vi "draw1.vi"(0 "new position":cluster{"x":i16, "y":i16}, 1 "L 1":dbl(slide)=80.0 scale=0.0..200.0, 2 "L 2":dbl(slide)=80.0 scale=0.0..200.0, 3 "Angle1":dbl(knob)=-45.83837436417874 scale=-90.0..90.0, 4 "Angle 2":dbl(knob)=-72.06882847083946 scale=-90.0..90.0, 5 "input pic in loop":picture, 7 "bias":dbl) -> (14 "end effector":cluster{dbl, dbl}={159.01647214211073, 1.9100783062530127} {"?" format="%.1f"; "?" format="%#.1f"}, 15 "mag":dbl, 16 "angle":dbl, 17 "2D Picture":picture, 18 "shift pic":picture)   [LabVIEW 2024]
panel:
  # "A 2"
  # "L1"
  # "L2"
  # "A 1"
  # "mm"
  # "mm"
  # "mm"
  # "mm"
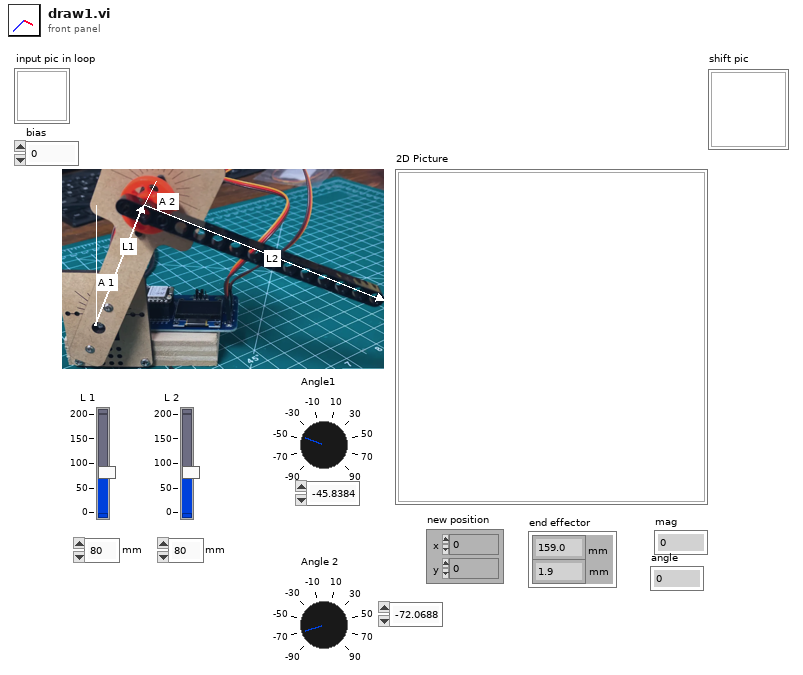
[diagram p1: front panel]
types:
  T1 = cluster{"Width":u16, "Style":enum32{"Solid", "Dash", "Dot", "DashDot", "DashDotDot"}}
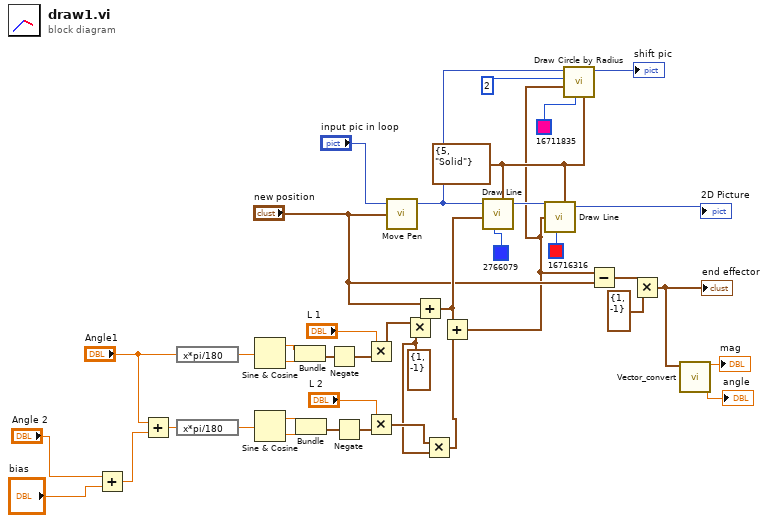
[diagram p0: block diagram]
diagram:
  w1 = cluster{"x":i16, "y":i16} {"x"=1, "y"=-1} ("new position")
  w15 = T1 {"Width"=5, "Style"=enum."Solid"} ("pen")
  n1 = Add(x="Angle 2", y="bias") -> (x+y=w8:dbl)
  n2 = Add(x="Angle1", y=w8) -> (x+y=w32:dbl)
  n3 = expression code="x*pi/180"("Angle1") -> (w40:dbl)
  n4 = expression code="x*pi/180"(w32) -> (w37:dbl)
  n5 = Sine & Cosine(0:w40) -> (1:w25:dbl, 2:w24:dbl)
  n6 = Sine & Cosine(0:w37) -> (1:w22:dbl, 2:w21:dbl)
  n7 = Bundle(w25, w24) -> (w39:cluster{dbl, dbl})  [unwired: 1 in]
  n8 = Bundle(w22, w21) -> (w38:cluster{dbl, dbl})  [unwired: 1 in]
  n9 = Negate(x=w39) -> (-x=w23:cluster{dbl, dbl})
  n10 = Negate(x=w38) -> (-x=w20:cluster{dbl, dbl})
  n11 = Multiply(x="L 1", y=w23) -> (x*y=w5:cluster{dbl, dbl})
  n12 = Multiply(x="L 2", y=w20) -> (x*y=w2:cluster{dbl, dbl})
  n13 = call <vilib>:"Move Pen.vi"("new position"="new position", "picture"="input pic in loop") -> ("new picture"=w13:picture)  [unwired: 3 in]
  n14 = Multiply(x=w5, y=w1) -> (x*y=w4:cluster{dbl, dbl})
  n15 = Add(x="new position", y=w4) -> (x+y=w35:cluster{dbl, dbl})
  n16 = Multiply(x=w2, y=w1) -> (x*y=w3:cluster{dbl, dbl})
  n17 = Add(x=w3, y=w35) -> (x+y=w14:cluster{dbl, dbl})
  n18 = call <vilib>:"Draw Line.vi"("picture"=w13, "end point"=w35, "color(black)"=u32 2766079, "pen"=w15) -> ("new picture"=w36:picture)  [unwired: 5 in]
  n19 = call <vilib>:"Draw Line.vi"("picture"=w36, "end point"=w14, "color(black)"=u32 16716316, "pen"=w15) -> ("new picture"=→"2D Picture":picture)  [unwired: 5 in]
  n20 = call <vilib>:"Draw Circle by Radius.vi"("pen"=w15, "color(black)"=u32 16711835, "pixel center"=w14, "radius"=u16 2 ("Width"), "picture"=w13) -> ("new picture"=→"shift pic":picture)  [unwired: 6 in]
  n21 = Subtract(x=w14, y="new position") -> (x-y=w28:cluster{dbl, dbl})
  n22 = Multiply(x=w28, y=cluster{"x":i16, "y":i16} {"x"=1, "y"=-1} ("new position")) -> (x*y=w19:cluster{dbl, dbl})
  "end effector" <- w19
  n23 = call "Vector_convert.vi"("x,y"=w19) -> ("angle"=→"angle":dbl, "mag"=→"mag":dbl)  [unwired: 9 in]
